vi "Config Set Get Tester.vi"   [LabVIEW 2014]
uses:
  DriverMasterSync/build/DriverMasterSync.lvlibp/Modules/HAL/DriverMasterSync/DriverMasterSyncClass/DriverMasterSync.lvclass
  <vilib>/Utility/LVLibp/NI_PackedLibraryUtility.lvlib
types:
  T1 = enum16{"open", "replace", "create", "open or create", "replace or create", "replace or create with confirmation"}
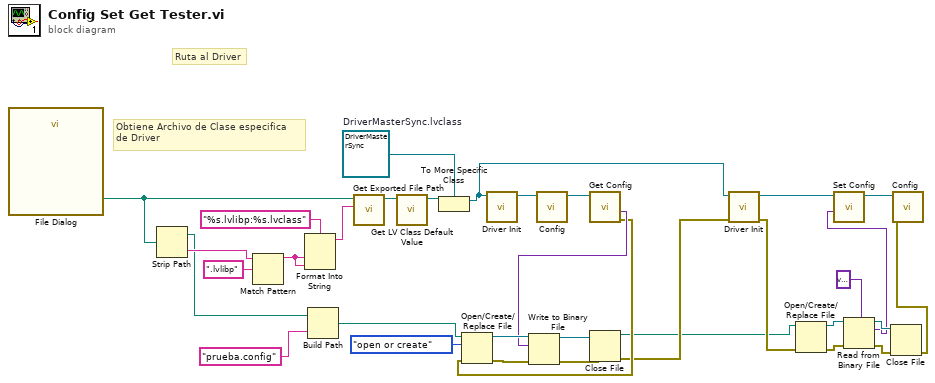
[diagram p0: block diagram]
diagram:
  w23 = refnum<class "DriverMasterSync.lvclass"> refnum  # DriverMasterSync.lvclass
  # "Ruta al Driver"
  # "Obtiene Archivo de Clase especifica\nde Driver"
  n1 = call "File Dialog"() -> ("selected path"=w27:path)  [unwired: 12 in, 3 out]
  n2 = Strip Path(path=w27) -> (stripped path=w21:path, name=w29:string)
  n3 = Match Pattern(string=w29, regular expression=".lvlibp") -> (before substring=w28:string)  [unwired: 1 in, 3 out]
  n4 = Format Into String(format string="%s.lvlibp:%s.lvclass", w28, w28) -> (resulting string=w33:string)  [unwired: 2 in, 1 out]
  n5 = Build Path(base path=w21, name or relative path="prueba.config" ("regular expression")) -> (appended path=w19:path)
  n6 = call <vilib>:"Get Exported File Path.vi"("qualified name"=w33, "packed library path"=w27) -> ("path"=w34:path)  [unwired: 8 in, 1 out]
  n7 = call <vilib>:"Get LV Class Default Value.vi"("class path"=w34) -> ("object"=w32:refnum<class>)  [unwired: 9 in, 1 out]
  n8 = To More Specific Class(target class=w23, reference=w32) -> (specific class reference=w15:refnum<class "DriverMasterSync.lvclass">)  [unwired: 1 in, 1 out]
  n9 = call-dynamic "Driver Init.vi"("DriverMasterSync in"=w15) -> ("DriverMasterSync out"=w24:refnum<class "DriverMasterSync.lvclass">)  [unwired: 9 in, 1 out]
  n10 = call-dynamic "Config.vi"("DriverMasterSync in"=w24) -> ("DriverMasterSync out"=w26:refnum<class "DriverMasterSync.lvclass">)  [unwired: 8 in, 2 out]
  n11 = call-dynamic "Get Config.vi"("DriverMasterSync in"=w26) -> ("error out"=w4:errorcluster, "Config Data"=w16:variant)  [unwired: 8 in, 1 out]
  n12 = Open/Create/Replace File(file path (use dialog)=w19, error in=w4, operation (0:open)=T1."open or create") -> (refnum out=w17:refnum<file>, error out=w12:errorcluster)  [unwired: 3 in, 1 out]
  n13 = Write to Binary File(file (use dialog)=w17, data=w16, error in=w12) -> (refnum out=w13:refnum<file>, error out=w11:errorcluster)  [unwired: 3 in, 1 out]
  n14 = Close File(refnum=w13, error in=w11) -> (path=w1:path, error out=w3:errorcluster)
  n15 = call-dynamic "Driver Init.vi"("error in (no error)"=w3, "DriverMasterSync in"=w15) -> ("error out"=w5:errorcluster, "DriverMasterSync out"=w14:refnum<class "DriverMasterSync.lvclass">)  [unwired: 8 in]
  n16 = Open/Create/Replace File(file path (use dialog)=w1, error in=w5) -> (refnum out=w10:refnum<file>, error out=w22:errorcluster)  [unwired: 4 in, 1 out]
  n17 = Read from Binary File(5:variant, 8:w22, 11:w10) -> (0:w8:errorcluster, 2:w6:variant, 3:w9:refnum<file>)  [unwired: 3 in, 1 out]
  n18 = call-dynamic "Set Config.vi"("Config Data"=w6, "DriverMasterSync in"=w14) -> ("DriverMasterSync out"=w25:refnum<class "DriverMasterSync.lvclass">)  [unwired: 8 in, 1 out]
  n19 = Close File(refnum=w9, error in=w8) -> (error out=w2:errorcluster)  [unwired: 1 out]
  n20 = call-dynamic "Config.vi"("error in (no error)"=w2, "DriverMasterSync in"=w25) -> ()  [unwired: 7 in, 3 out]
